vi "Label_Answer_Window_Logging.vi"(11 "rt fifo":refnum<k33>) -> ()   [LabVIEW 2020]
uses:
  Global Variables/Time_Trigger.vi
  Global Variables/Global Label.vi
  Global Variables/Global User_Answer.vi
  Global Variables/Window_Size.vi
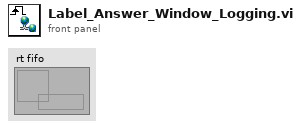
[diagram p1: front panel]
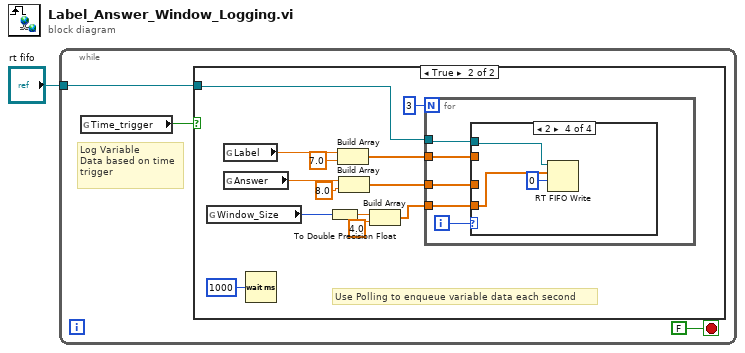
[diagram p0: block diagram]
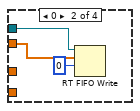
[diagram p4: hidden frame]
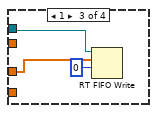
[diagram p5: hidden frame]
diagram:
  n1 = while {
    tunnel: "rt fifo" -> [w2]
    stop <- FALSE stop-if-true
    # "Log Variable \nData based on time\ntrigger"
    n2 = global read "Time_Trigger.vi" "Time_trigger"() -> (w3:bool)
    n3 = case shown="True" w3 {
      tunnel: w2 -> [_ w11]
      frame False {
      }
      frame True {
        # "Use Polling to enqueue variable data each second"
        n4 = global read "Window_Size.vi" "Window_Size"() -> (w14:i64)
        n5 = global read "Global Label.vi" "Label"() -> (w17:dbl)
        n6 = global read "Global User_Answer.vi" "Answer"() -> (w15:dbl)
        n7 = Wait (ms)(milliseconds to wait=u32 1000) -> ()  [unwired: 1 out]
        n8 = To Double Precision Float(number=w14) -> (double precision float=w13:dbl)
        n9 = Build Array(w17, 7.0 ("element")) -> (w6:dbl[])
        n10 = Build Array(w15, 8.0 ("element")) -> (w7:dbl[])
        n11 = Build Array(w13, 4.0) -> (w8:dbl[])
        n12 = for {
          N: 3 -> [_]
          tunnel: w11 -> [w22]
          tunnel: w8 -> [w19]
          tunnel: w7 -> [w18]
          tunnel: w6 -> [w20]
          i -> [w21]
          n13 = case shown="2" w21 {
            tunnel: w22 -> [_ w25 w28 w31]
            tunnel: w20 -> [_ w24 _ _]
            tunnel: w19 -> [_ _ _ w30]
            tunnel: w18 -> [_ _ w27 _]
            frame Default {
            }
            frame 0 {
              n14 = RT FIFO Write(0:w25, 1:w24, 2:0 ("timeout in ms (0)")) -> ()  [unwired: 2 in, 4 out]
            }
            frame 1 {
              n15 = RT FIFO Write(0:w28, 1:w27, 2:0 ("timeout in ms (0)")) -> ()  [unwired: 2 in, 4 out]
            }
            frame 2 {
              n16 = RT FIFO Write(0:w31, 1:w30, 2:0 ("timeout in ms (0)")) -> ()  [unwired: 2 in, 4 out]
            }
          }
        }
      }
    }
  }
